vi "Find Nodes Attribute.vi"(8 "error in":errorcluster, 10 "XPath":T1, 11 "Node in":refnum<k20>) -> (0 "error out":errorcluster, 2 "Attribute":string[](array[string]), 3 "Node out":refnum<k20>)   [LabVIEW 2020, in "VI Properties Editor.lvlib"]
uses:
  VI Properties Editor.lvlib
  <vilib>/xml/NI_XML.lvlib
  <resource>/objmgr/DOMUserDefRef.rc
  CTLs/XPath Get Attribute.ctl
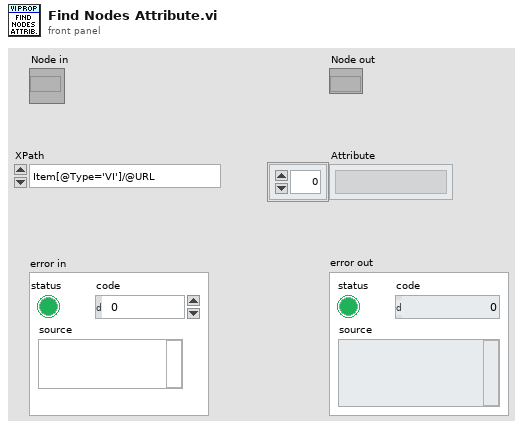
[diagram p1: front panel]
types:
  T1 = typedef "VI Properties Editor.lvlib/XPath Get Attribute.ctl" = enum16{"Item[@Type='VI']/@URL", "Item[@Type='LVClass']/@URL", "Item[@Type='Library']/@URL", "Item[@Type='Folder' and not (@URL)]/@Name", "@Name"}
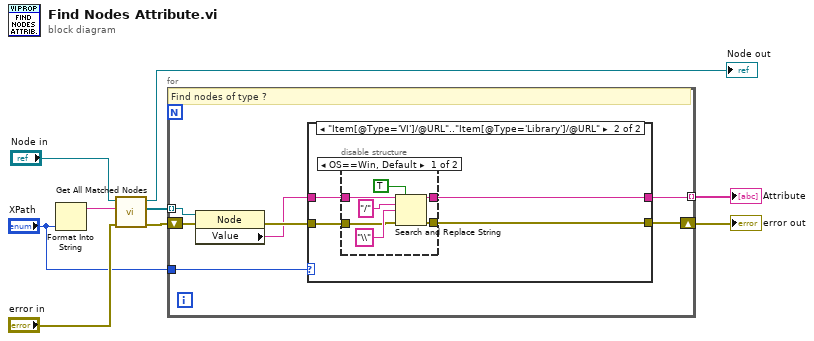
[diagram p0: block diagram]
diagram:
  n1 = Format Into String("XPath") -> (resulting string=w6:string)  [unwired: 3 in, 1 out]
  n2 = call <vilib>:"Get All Matched Nodes.vi"("error in (no error)"="error in", "XPath expression"=w6, "node in"="Node in") -> ("error out"=w8:errorcluster, "node result array"=w9:refnum<k20>[], "node out"=→"Node out":refnum<k20>)  [unwired: 6 in]
  n3 = for {
    tunnel: w9 -> [w15] mode=indexing
    tunnel: [w14] -> w7 mode=indexing
    shift-right: [w13] -> w3
    shift-left: w8 -> [w16]
    tunnel: "XPath" -> [w10]
    # "Find nodes of type ?"
    n4 = property class="Node"(reference=w15, error in=w16) -> (error out=w12:errorcluster, "Value"=w11:string)  [unwired: 1 out]
    n5 = case shown="\"Item[@Type='VI']/@URL\"..\"Item[@Type='Library']/@URL\"" w10 {
      tunnel: [w17 w22] -> w14
      tunnel: [w18 w21] -> w13
      tunnel: w12 -> [w18 w20]
      tunnel: w11 -> [w17 w19]
      frame "@Name", Default {
      }
      frame "Item[@Type='VI']/@URL".."Item[@Type='Library']/@URL" {
        n6 = disable-structure shown="OS==Win, Default" {
          disable-tunnel: [w29 w31] -> w22
          disable-tunnel: w19 -> [w28 w31]
          disable-tunnel: w20 -> [w24 w30]
          disable-tunnel: [w23 w30] -> w21
          frame condition #0 (active) {
            n7 = Search and Replace String(replace all?=TRUE ("replace all? (F)"), input string=w28, search string="/", replace string="\\" ("replace string (\"\")"), error in=w24) -> (result string=w29:string, error out=w23:errorcluster)  [unwired: 3 in, 2 out]
          }
          frame condition #1 {
          }
        }
      }
    }
  }
  "Attribute" <- w7
  "error out" <- w3
